vi "Write Runstate.vi"   [LabVIEW 2023, in "Cycler.lvclass"]
uses:
  Cycler.lvclass
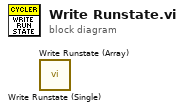
[diagram p0: block diagram]
diagram:
  n1 = call "Write Runstate (Single).vi"() -> ()  [unwired: 10 in, 2 out]
  n2 = call "Write Runstate (Array).vi"() -> ()  [unwired: 10 in, 2 out]
